vi "Read Error Handling Parameters.vi"(4 "Error In":errorcluster, 7 "Text in":refnum<class "Config Data_Text.lvclass">) -> (0 "Error Out":errorcluster, 1 "Buttons":T1, 2 "Action":T2(ring)=enum."Ok Only", 3 "Text out":refnum<class "Config Data_Text.lvclass">)   [LabVIEW 2014, in "Config Data.lvlib" / "Config Data_Text.lvclass"]
uses:
  Config Data_Text.lvclass
  <vilib>/Utility/config.llb/Read Key (String).vi
  <vilib>/Utility/config.llb/Write Key (String).vi
  <vilib>/Utility/config.llb/NI_LVConfig.lvlib
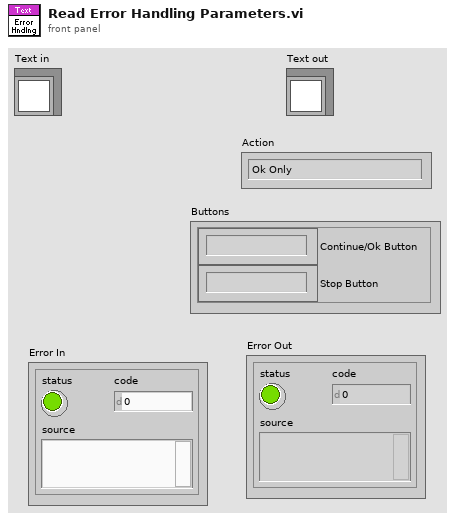
[diagram p1: front panel]
types:
  T1 = cluster{"Continue/Ok Button":string, "Stop Button":string}
  T2 = enum16{"Ok + Logging", "Continue/Stop + Logging", "Logging Only", "Ok Only", "Continue/Stop Only"}
  T3 = typedef "NI_LVConfig.lvlib/Config Data RefNum.ctl" = refnum<k1>
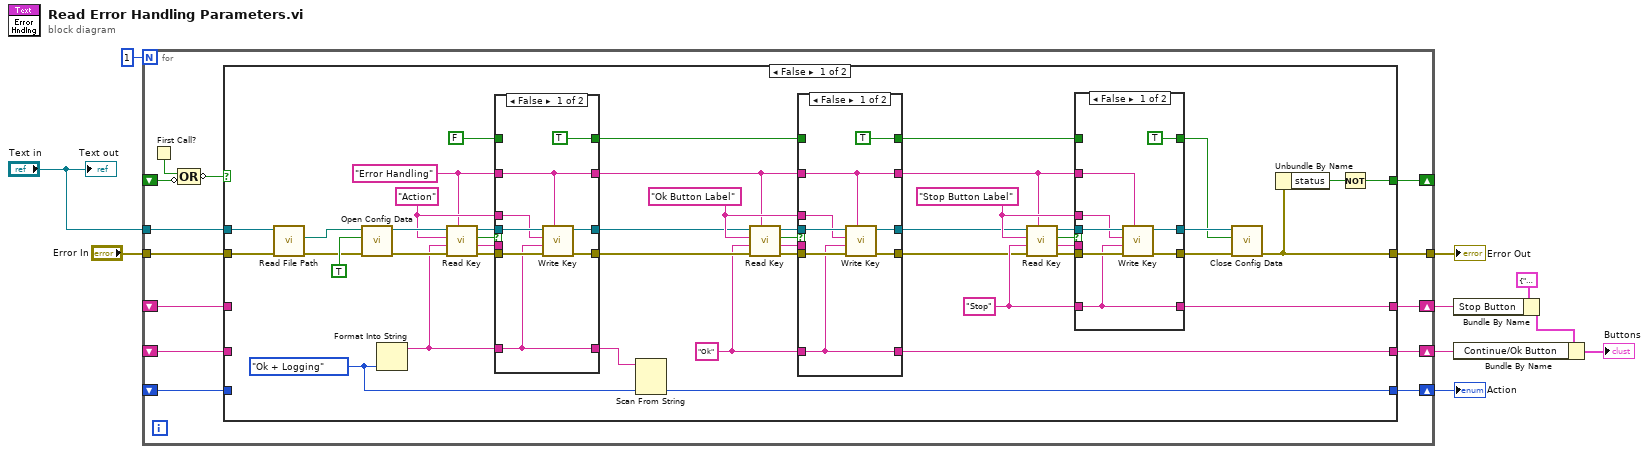
[diagram p0: block diagram]
diagram:
  n1 = for {
    N: 1 -> [_]
    tunnel: [w23] -> w7
    tunnel: "Error In" -> [w22]
    shift-right: [w21] -> _
    shift-left: _ -> [w20]
    shift-right: [w17] -> w6
    shift-left: _ -> [w16]
    shift-right: [w15] -> w2
    shift-left: _ -> [w14]
    shift-right: [w13] -> w5
    shift-left: _ -> [w12]
    tunnel: "Text in" -> [w11]
    n2 = First Call?() -> (First Call?: T/F=w18:bool)
    n3 = Compound Arithmetic op=OR(w18, invert w20) -> (invert w19:bool)
    n4 = case shown="False" w19 {
      selector: w19 -> [_ w111]
      tunnel: w22 -> [w27 w112]
      tunnel: [w57 w112] -> w23
      tunnel: [w59 w111] -> w21
      tunnel: [w54 w110] -> w17
      tunnel: w16 -> [_ w110]
      tunnel: [w42 w109] -> w15
      tunnel: w14 -> [_ w109]
      tunnel: [w30 w108] -> w13
      tunnel: w12 -> [_ w108]
      tunnel: w11 -> [w24 _]
      frame False {
        w41 = "Stop" ("default value")
        w37 = "Stop Button Label" ("default value")
        w43 = "Ok" ("default value")
        w51 = "Ok Button Label" ("default value")
        w53 = T2."Ok + Logging" ("Action")
        w58 = "Error Handling" ("default value")
        w63 = "Action" ("default value")
        n5 = call "Read File Path.vi"("Error In"=w27, "Text In"=w24) -> ("Error Out"=w26:errorcluster, "File Path"=w25:path)  [unwired: 3 in, 1 out]
        n6 = call <vilib>:"Open Config Data.vi"("error in (no error)"=w26, "create file if necessary (T)"=TRUE ("create file if necessary? (T)"), "configuration file path"=w25) -> ("error out"=w68:errorcluster, "refnum"=w67:T3)  [unwired: 6 in, 1 out]
        n7 = Format Into String(w53) -> (resulting string=w56:string)  [unwired: 3 in, 1 out]
        n8 = call-poly <vilib>:"Read Key.vi"("section"=w58, "error in (no error)"=w68, "default value"=w56, "key"=w63, "refnum"=w67) -> ("error out"=w64:errorcluster, "value"=w62:string, "found?"=w66:bool, "refnum out"=w65:T3)  [unwired: 1 in, 2 out]
        n9 = case shown="False" w66 {
          tunnel: w65 -> [w101 w106]
          tunnel: w58 -> [w95 w103]
          tunnel: w64 -> [w102 w107]
          tunnel: [w98 w107] -> w46
          tunnel: [w99 w106] -> w47
          tunnel: w63 -> [w100 _]
          tunnel: w62 -> [_ w105]
          tunnel: [w96 w105] -> w55
          tunnel: FALSE ("write configuration file? (T)") -> [_ w104]
          tunnel: [TRUE ("write configuration file? (T)") w104] -> w44
          tunnel: w56 -> [w96 _]
          tunnel: [w95 w103] -> w45
          frame False {
            n10 = call-poly <vilib>:"Write Key.vi"("section"=w95, "error in (no error)"=w102, "value"=w96, "key"=w100, "refnum"=w101) -> ("error out"=w98:errorcluster, "refnum out"=w99:T3)  [unwired: 1 in, 4 out]
          }
          frame True {
          }
        }
        n11 = Scan From String(input string=w55, default 1=w53) -> (output 1=w54:T2)  [unwired: 3 in, 3 out]
        n12 = call-poly <vilib>:"Read Key.vi"("section"=w45, "error in (no error)"=w46, "default value"=w43, "key"=w51, "refnum"=w47) -> ("error out"=w50:errorcluster, "value"=w52:string, "found?"=w48:bool, "refnum out"=w49:T3)  [unwired: 1 in, 2 out]
        n13 = case shown="False" w48 {
          tunnel: w49 -> [w88 w93]
          tunnel: w45 -> [w82 w90]
          tunnel: w50 -> [w89 w94]
          tunnel: [w85 w94] -> w31
          tunnel: [w86 w93] -> w32
          tunnel: w51 -> [w87 _]
          tunnel: w52 -> [_ w92]
          tunnel: [w83 w92] -> w42
          tunnel: w44 -> [_ w91]
          tunnel: [TRUE ("write configuration file? (T)") w91] -> w29
          tunnel: w43 -> [w83 _]
          tunnel: [w82 w90] -> w33
          frame False {
            n14 = call-poly <vilib>:"Write Key.vi"("section"=w82, "error in (no error)"=w89, "value"=w83, "key"=w87, "refnum"=w88) -> ("error out"=w85:errorcluster, "refnum out"=w86:T3)  [unwired: 1 in, 4 out]
          }
          frame True {
          }
        }
        n15 = call-poly <vilib>:"Read Key.vi"("section"=w33, "error in (no error)"=w31, "default value"=w41, "key"=w37, "refnum"=w32) -> ("error out"=w38:errorcluster, "value"=w36:string, "found?"=w40:bool, "refnum out"=w39:T3)  [unwired: 1 in, 2 out]
        n16 = case shown="False" w40 {
          tunnel: w39 -> [w76 w80]
          tunnel: w33 -> [w75 _]
          tunnel: w38 -> [w77 w81]
          tunnel: [w72 w81] -> w35
          tunnel: [w73 w80] -> w34
          tunnel: w37 -> [w74 _]
          tunnel: w36 -> [_ w79]
          tunnel: [w70 w79] -> w30
          tunnel: [TRUE ("write configuration file? (T)") w78] -> w28
          tunnel: w41 -> [w70 _]
          tunnel: w29 -> [_ w78]
          frame False {
            n17 = call-poly <vilib>:"Write Key.vi"("section"=w75, "error in (no error)"=w77, "value"=w70, "key"=w74, "refnum"=w76) -> ("error out"=w72:errorcluster, "refnum out"=w73:T3)  [unwired: 1 in, 4 out]
          }
          frame True {
          }
        }
        n18 = call <vilib>:"Close Config Data.vi"("error in (no error)"=w35, "write file if changed (T)"=w28, "refnum"=w34) -> ("error out"=w57:errorcluster)  [unwired: 8 out]
        n19 = Unbundle By Name(w57) -> ("status"=w60:bool)
        n20 = Not(x=w60) -> (.not. x?=w59:bool)
      }
      frame True {
      }
    }
  }
  "Error Out" <- w7
  "Action" <- w6
  n21 = Bundle By Name(cluster=T1 {"Continue/Ok Button"="Continue", "Stop Button"="Stop"} ("Buttons"), "Stop Button"=w5) -> (w3:T1)
  n22 = Bundle By Name(cluster=w3, "Continue/Ok Button"=w2) -> (→"Buttons":T1)
  "Text out" <- "Text in"
